vi "Timers.vi"(9 "Timer in":u32) -> (1 "Timer out":u32)   [LabVIEW 2016]
uses:
  Robot Global Data.vi
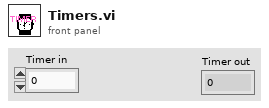
[diagram p1: front panel]
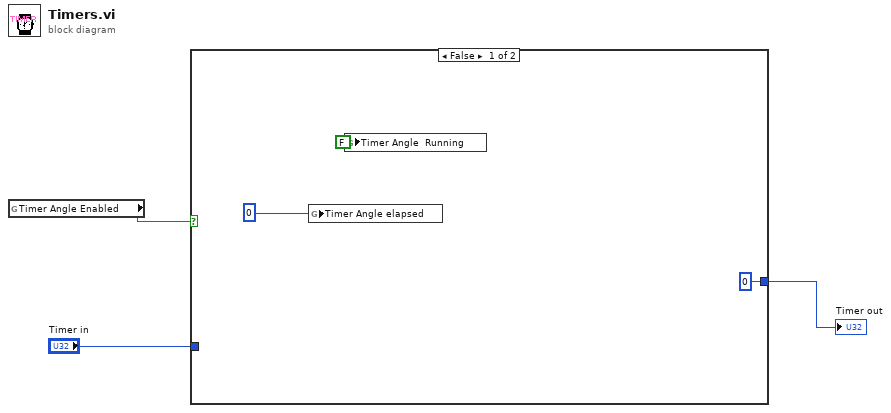
[diagram p0: block diagram]
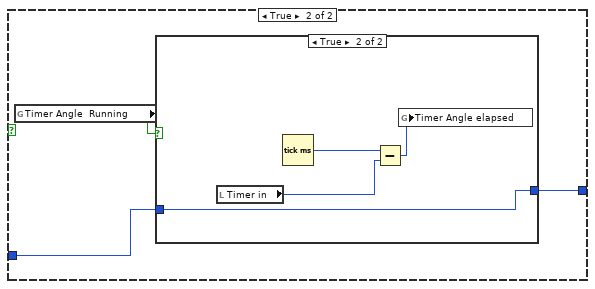
[diagram p2: hidden frame]
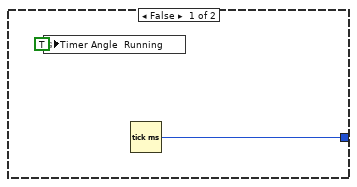
[diagram p3: hidden frame]
diagram:
  n1 = global read "Robot Global Data.vi" "Timer Angle Enabled"() -> (w3:bool)
  n2 = case shown="False" w3 {
    tunnel: [u32 0 ("millisecond timer value") w8] -> w2
    tunnel: "Timer in" -> [_ w7]
    frame False {
      n3 = global write "Robot Global Data.vi" "Timer Angle elapsed"(u32 0 ("Timer1 elapsed")) -> ()
      n4 = global write "Robot Global Data.vi" "Timer Angle  Running"(FALSE ("Timer1 Running")) -> ()
    }
    frame True {
      n5 = global read "Robot Global Data.vi" "Timer Angle  Running"() -> (w9:bool)
      n6 = case shown="True" w9 {
        tunnel: [w11 w12] -> w8
        tunnel: w7 -> [_ w12]
        frame False {
          n7 = global write "Robot Global Data.vi" "Timer Angle  Running"(TRUE ("Timer1 Running")) -> ()
          n8 = Tick Count (ms)() -> (millisecond timer value=w11:u32)
        }
        frame True {
          n9 = local read "Timer in"() -> (w14:u32)
          n10 = Tick Count (ms)() -> (millisecond timer value=w15:u32)
          n11 = Subtract(x=w15, y=w14) -> (x-y=w13:u32)
          n12 = global write "Robot Global Data.vi" "Timer Angle elapsed"(w13) -> ()
        }
      }
    }
  }
  "Timer out" <- w2
